vi "Toggle2 (SubVI).vi"(6 "HasPressedShifterButton":bool, 7 "Button 1":bool, 9 "Shifter On":bool, 10 "Shifter On 2":refnum<vi>, 11 "Boolean in":refnum<vi>) -> (3 "Shifter On out":bool)   [LabVIEW 2012]
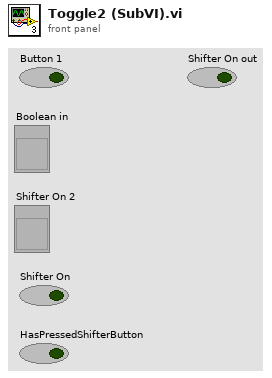
[diagram p1: front panel]
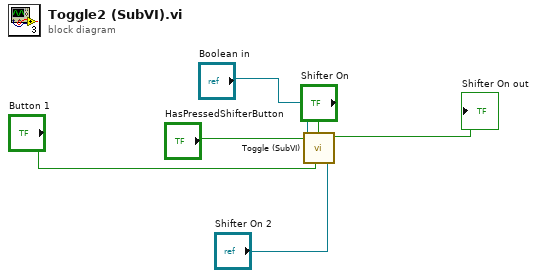
[diagram p0: block diagram]
diagram:
  n1 = call "Toggle (SubVI).vi"("Button 1"="Button 1", "Shifter On in"="Shifter On", "HasPressedShifterButton"="HasPressedShifterButton", "reference in"="Shifter On 2", "Boolean in"="Boolean in") -> ("Shifter On out"=→"Shifter On out":bool)  [unwired: 6 in]
